vi "Riffle Array (DBL).vi"(10 "seed":i32=-1, 11 "X":dbl[](array[numeric])) -> (0 "error":i32, 2 "Riffled Index":i32[](array[numeric]), 3 "Riffled {X}":dbl[](array[numeric]))   [LabVIEW 2018, in "NI_AALBase.lvlib"]
doc: "Riffles the elements in the input array <B>X</B>. Wire data to the <B>X</B> input to determine the polymorphic instance to use or manually select the instance."
uses:
  NI_AALBase.lvlib
  <resource>/lvanlys.dll
panel:
  # "Riffle Array (DBL)"
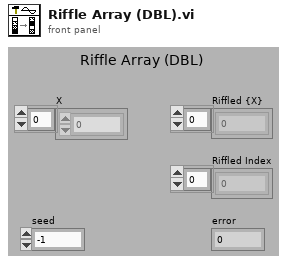
[diagram p1: front panel]
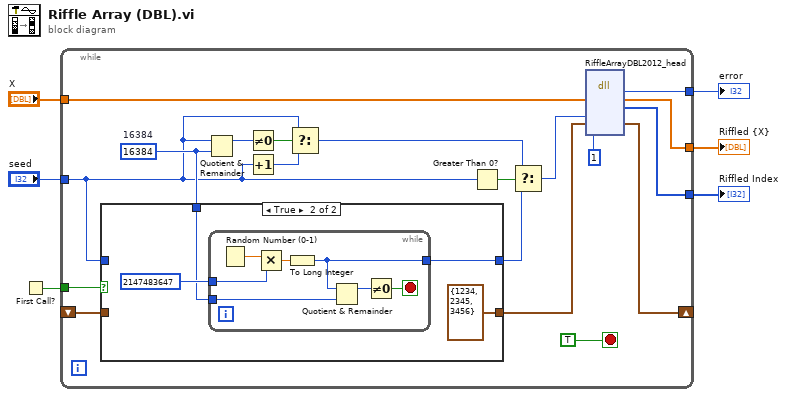
[diagram p0: block diagram]
diagram:
  n1 = First Call?() -> (First Call?: T/F=w6:bool)
  n2 = while {
    tunnel: "seed" -> [w8]
    shift-right: [w21] -> _
    shift-left: _ -> [w9]
    tunnel: w6 -> [w7]
    tunnel: [w24] -> w3
    tunnel: [w23] -> w5
    tunnel: "X" -> [w22]
    tunnel: [w20] -> w1
    stop <- TRUE stop-if-true
    w12 = 16384  # 16384
    n3 = case shown="True" w7 {
      tunnel: w9 -> [w27 _]
      tunnel: [w27 cluster{"xSeed":i32, "ySeed":i32, "zSeed":i32} {"xSeed"=1234, "ySeed"=2345, "zSeed"=3456} ("RNGState")] -> w10
      tunnel: [w26 w28] -> w13
      tunnel: w8 -> [w26 _]
      tunnel: w12 -> [_ w29]
      frame False {
      }
      frame True {
        n4 = while {
          tunnel: [w36] -> w28
          tunnel: w29 -> [w35]
          tunnel: 2147483647 ("x") -> [w32]
          stop <- w33 stop-if-true
          n5 = Random Number (0-1)() -> (number: 0 to 1=w37:dbl)
          n6 = Multiply(x=w37, y=w32) -> (x*y=w38:dbl)
          n7 = To Long Integer(number=w38) -> (32bit integer=w36:i32)
          n8 = Quotient & Remainder(x=w36, y=w35) -> (x-y*floor(x/y)=w34:i32)  [unwired: 1 out]
          n9 = Not Equal To 0?(x=w34) -> (x != 0?=w33:bool)
        }
      }
    }
    n10 = Quotient & Remainder(x=w8, y=w12) -> (x-y*floor(x/y)=w17:i32)  [unwired: 1 out]
    n11 = Not Equal To 0?(x=w17) -> (x != 0?=w16:bool)
    n12 = Increment(x=w8) -> (x+1=w15:i32)
    n13 = Select(t=w8, s=w16, f=w15) -> (s? t:f=w14:i32)
    n14 = Greater Than 0?(x=w8) -> (x > 0?=w18:bool)
    n15 = Select(t=w14, s=w18, f=w13) -> (s? t:f=w11:i32)
    n16 = dll-call lib="C:/Program Files (x86)/National Instruments/LabVIEW 2018/resource/lvanlys.*" fn="RiffleArrayDBL2012_head"("riffle"=w22, "seed"=w11, "rngState"=w10, "option"=1) -> ("return type"=w24:i32, "riffle"=w23:dbl[], "riffleIndex"=w20:i32[], "rngState"=w21:cluster{"xSeed":i32, "ySeed":i32, "zSeed":i32})  [unwired: 6 in, 2 out]
  }
  "Riffled {X}" <- w5
  "error" <- w3
  "Riffled Index" <- w1
